vi "UsrProfiles-Window-Save options.vi"(7 "Colour":u32(colorbox)=16777225) -> (0 "error out":errorcluster, 1 "Cancelled":bool)   [LabVIEW 2013]
doc: "Use this template to create a dialog box with event handling."
uses:
  Typedefs/Changed parameter cluster.ctl
  <vilib>/Utility/miscctls.llb/LVPointTypeDef.ctl
  Global Variables/General Globals.vi
panel:
  in  "Changes array ctrl":T1[](array[typedef])
  in  "Cancel":bool
  in  "Save":bool
  # "Parameter"
  # "Old value"
  # "New value"
  # "Save?"
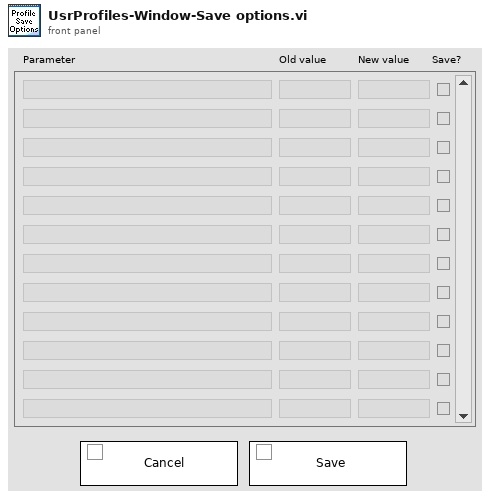
[diagram p1: front panel]
types:
  T1 = typedef "Changed parameter cluster.ctl" = cluster{"Name":string, "Old value":string, "New value":string, "Save":bool}
  T2 = typedef "LVPointTypeDef.ctl" = cluster{"Horizontal":i16, "Vertical":i16}
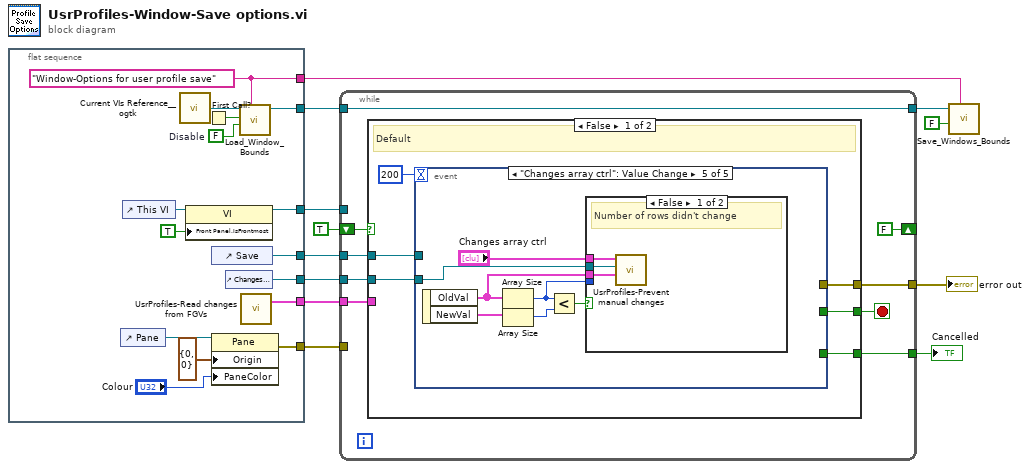
[diagram p0: block diagram]
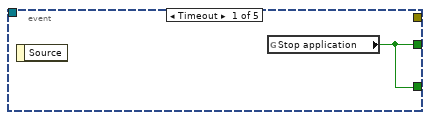
[diagram p2: hidden frame]
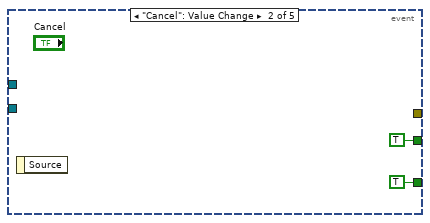
[diagram p3: hidden frame]
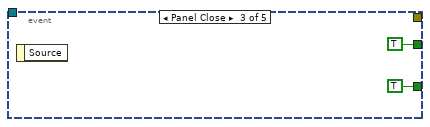
[diagram p4: hidden frame]
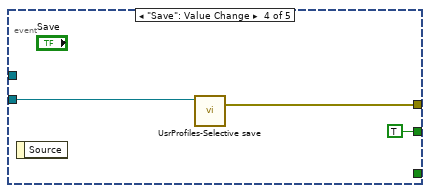
[diagram p5: hidden frame]
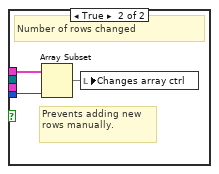
[diagram p6: hidden frame]
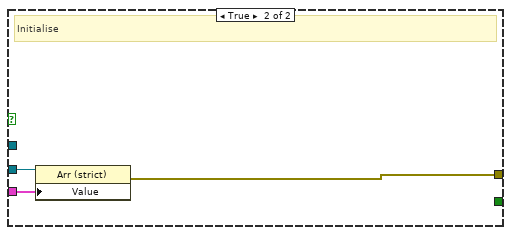
[diagram p7: hidden frame]
diagram:
  n1 = flat-sequence {
    tunnel: [w25] -> w12
    tunnel: [w23] -> w11
    tunnel: [w18] -> w10
    tunnel: [w17] -> w8
    tunnel: [w15] -> w6
    tunnel: [w14] -> w4
    tunnel: [w13] -> w1
    frame #0 {
      w19 = FALSE  # Disable
      w18 = "Window-Options for user profile save" ("Window Name (i.e. Key)")
      n2 = control-ref of="Pane"() -> (w22:refnum<vi>)
      n3 = control-ref of="This VI"() -> (w26:refnum<vi>)
      n4 = call "Current VIs Reference__ogtk.vi"() -> ("Current VI's reference"=w21:refnum<vi>)  [unwired: 5 in]
      n5 = property on="Property Node" class="VI"(reference=w26, "Front Panel.IsFrontmost"=TRUE ("Front Panel Window:Is Frontmost")) -> (reference out=w25:refnum<vi>)  [unwired: 1 in, 1 out]
      n6 = First Call?() -> (First Call?: T/F=w20:bool)
      n7 = control-ref of="Save"() -> (w15:refnum<vi>)
      n8 = property class="Pane"(reference=w22, "Origin"=T2 {"Horizontal"=0, "Vertical"=0}, "PaneColor"="Colour") -> (error out=w23:errorcluster)  [unwired: 1 in, 1 out]
      n9 = control-ref of="Changes array ctrl"() -> (w14:refnum<vi>)
      n10 = call "Load_Window_Bounds.vi"("Window Name (i.e. Key)"=w18, "Disable"=w19, "First Call"=w20, "Window VI's Ref"=w21) -> ("reference out"=w17:refnum<vi>)  [unwired: 4 in, 3 out]
      n11 = call "UsrProfiles-Read changes from FGVs.vi"() -> ("All changed parameters info"=w13:T1[])  [unwired: 10 in, 5 out]
    }
  }
  n12 = while {
    tunnel: w11 -> [_]
    tunnel: w12 -> [_]
    tunnel: [w35] -> w5
    tunnel: w8 -> [w34]
    tunnel: [w34] -> w7
    tunnel: w6 -> [w33]
    tunnel: w4 -> [w32]
    shift-right: [FALSE] -> _
    shift-left: TRUE -> [w31]
    tunnel: [w29] -> w2
    tunnel: w1 -> [w28]
    stop <- w36 stop-if-true
    n13 = case shown="False" w31 {
      tunnel: [w42 _] -> w36
      tunnel: [w40 _] -> w35
      tunnel: w33 -> [w39 _]
      tunnel: w32 -> [w38 w66]
      tunnel: [w37 w65] -> w29
      tunnel: w28 -> [_ w64]
      frame False {
        # "Default"
        n14 = event shown="[4] \"Changes array ctrl\": Value Change" {
          selector: _ -> [_ _ _ _ _]
          dyn-events: _ -> [_ _ _ _ _]
          timeout: 200 -> [_ _ _ _ _]
          tunnel: [w43 TRUE ("Stop?") TRUE ("Stop?") TRUE ("Stop?") _] -> w42
          tunnel: [w43 TRUE ("Stop subpanel") TRUE ("Stop subpanel") _ _] -> w40
          tunnel: w39 -> [_ _ _ _ _]
          tunnel: w38 -> [_ _ _ w49 w51]
          tunnel: [_ _ _ w48 _] -> w37
          event Timeout {
            n15 = event-data() -> ()  [unwired: 1 in, 1 out]
            n16 = global read "General Globals.vi" "Stop application"() -> (w43:bool)
          }
          event "Cancel": Value Change {
            n17 = event-data() -> ()  [unwired: 1 in, 1 out]
          }
          event Panel Close {
            n18 = event-data() -> ()  [unwired: 1 in, 1 out]
          }
          event "Save": Value Change {
            n19 = event-data() -> ()  [unwired: 1 in, 1 out]
            n20 = call "UsrProfiles-Selective save.vi"("Changes array ctrl"=w49) -> ("error out"=w48:errorcluster)  [unwired: 10 in]
          }
          event "Changes array ctrl": Value Change {
            n21 = event-data() -> ("OldVal"=w52:T1[], "NewVal"=w57:T1[])  [unwired: 1 in]
            n22 = Array Size(array=w52) -> (size(s)=w53:i32)
            n23 = Array Size(array=w57) -> (size(s)=w56:i32)
            n24 = Less?(x=w53, y=w56) -> (x < y?=w55:bool)
            n25 = case shown="False" w55 {
              tunnel: "Changes array ctrl" -> [w58 w63]
              tunnel: w53 -> [_ w62]
              tunnel: w52 -> [w60 _]
              tunnel: w51 -> [w59 _]
              frame False {
                # "Number of rows didn't change"
                n26 = call "UsrProfiles-Prevent manual changes.vi"("Changes array ctrl (Old value)"=w60, "Changes array ctrl"=w59, "Changes array ctrl (New value)"=w58) -> ()  [unwired: 8 in, 1 out]
              }
              frame True {
                # "Prevents adding new rows manually."
                # "Number of rows changed"
                n27 = Array Subset(array=w63, length=w62) -> (w61:T1[])  [unwired: 1 in]
                n28 = local write "Changes array ctrl"(w61) -> ()
              }
            }
          }
        }
      }
      frame True {
        # "Initialise"
        n29 = property class="Arr (strict)"(reference=w66, "Value"=w64) -> (error out=w65:errorcluster)  [unwired: 1 in, 1 out]
      }
    }
  }
  "Cancelled" <- w5
  "error out" <- w2
  n30 = call "Save_Windows_Bounds.vi"("Window Name (i.e. Key)"=w10, "Front Panel Window:Open"=FALSE, "Window VI's Ref"=w7) -> ()  [unwired: 8 in, 1 out]
